vi "Read Sample Parameters.vi"(8 "error in":errorcluster, 11 "TDMS in":refnum<class "TDMS.lvclass">) -> (0 "error out":errorcluster, 1 "sample params":variant[][](array[variant]), 2 "sample param names":string[](array[string]), 3 "TDMS out":refnum<class "TDMS.lvclass">)   [LabVIEW 2011, in "TDMS.lvclass"]
uses:
  TDMS.lvclass
  TDMS.lvclass/TDMS.ctl
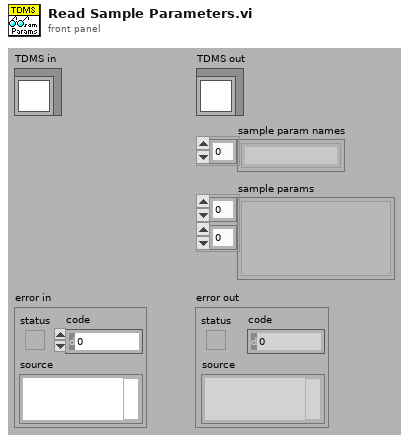
[diagram p1: front panel]
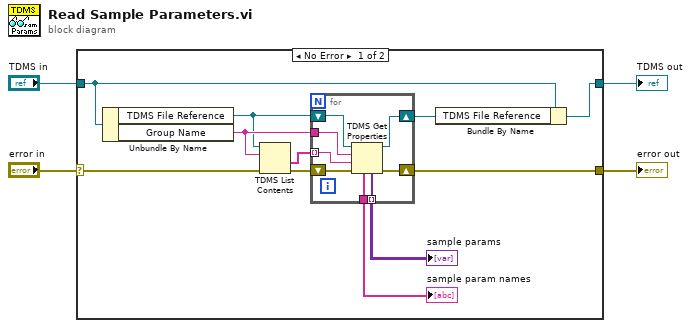
[diagram p0: block diagram]
diagram:
  n1 = case shown="No Error" "error in" {
    selector: "error in" -> [w14 w24]
    tunnel: [w6 w24] -> w1
    tunnel: [w7 w25] -> w2
    tunnel: "TDMS in" -> [w9 w25]
    frame No Error {
      n2 = Unbundle By Name(w9) -> ("TDMS File Reference"=w12:refnum<k34>, "Group Name"=w13:string)
      n3 = TDMS List Contents(4:w14, 6:w13, 7:w12) -> (0:w11:errorcluster, 1:w10:string[])  [unwired: 2 out]
      n4 = for {
        tunnel: [w23] -> w15
        tunnel: w13 -> [w22]
        shift-right: [w18] -> w6
        shift-left: w11 -> [w20]
        tunnel: w10 -> [w19] mode=indexing
        shift-right: [w17] -> w8
        shift-left: w12 -> [w21]
        tunnel: [w16] -> w5 mode=indexing
        n5 = TDMS Get Properties(8:w20, 9:w19, 10:w22, 11:w21) -> (0:w18:errorcluster, 3:w17:refnum<k34>, 4:w16:variant[], 6:w23:string[])  [unwired: 2 in, 2 out]
      }
      "sample params" <- w5
      "sample param names" <- w15
      n6 = Bundle By Name(cluster=w9, "TDMS File Reference"=w8) -> (w7:refnum<class "TDMS.lvclass">)
    }
    frame Error {
    }
  }
  "error out" <- w1
  "TDMS out" <- w2
